vi "get Object By Name.vi"(10 "Name":string, 11 "Scene in":refnum<class "Scene.lvclass">) -> (2 "Index":i32, 3 "Object":T1 {"Triangles"."Vertex 3"."UV"."v" min=0 max=1 step=0.1; "Triangles"."Vertex 3"."UV"."u" min=0 max=1 step=0.1; "Triangles"."Vertex 2"."UV"."v" min=0 max=1 step=0.1; "Triangles"."Vertex 2"."UV"."u" min=0 max=1 step=0.1; "Triangles"."Vertex 1"."UV"."v" min=0 max=1 step=0.1; "Triangles"."Vertex 1"."UV"."u" min=0 max=1 step=0.1})   [LabVIEW 2020, in "Scene.lvclass"]
uses:
  Scene.lvclass
  Scene.lvclass/Scene.ctl
  Graphics/Libraries/3D/Vector 3D.ctl
  Graphics/Libraries/3D/3D.lvlib
  Graphics/Libraries/3D/Transform.ctl
  Graphics/Libraries/3D/Object.ctl
  Graphics/Libraries/Raster/UV.ctl
  Graphics/Libraries/Raster/Raster.lvlib
  Graphics/Libraries/3D/Vertex.ctl
  Graphics/Libraries/3D/Triangle.ctl
  Graphics/Libraries/Raster/Rectangle Dimensions.ctl
  Graphics/Libraries/Raster/Texture.ctl
  Graphics/Libraries/3D/Material.ctl
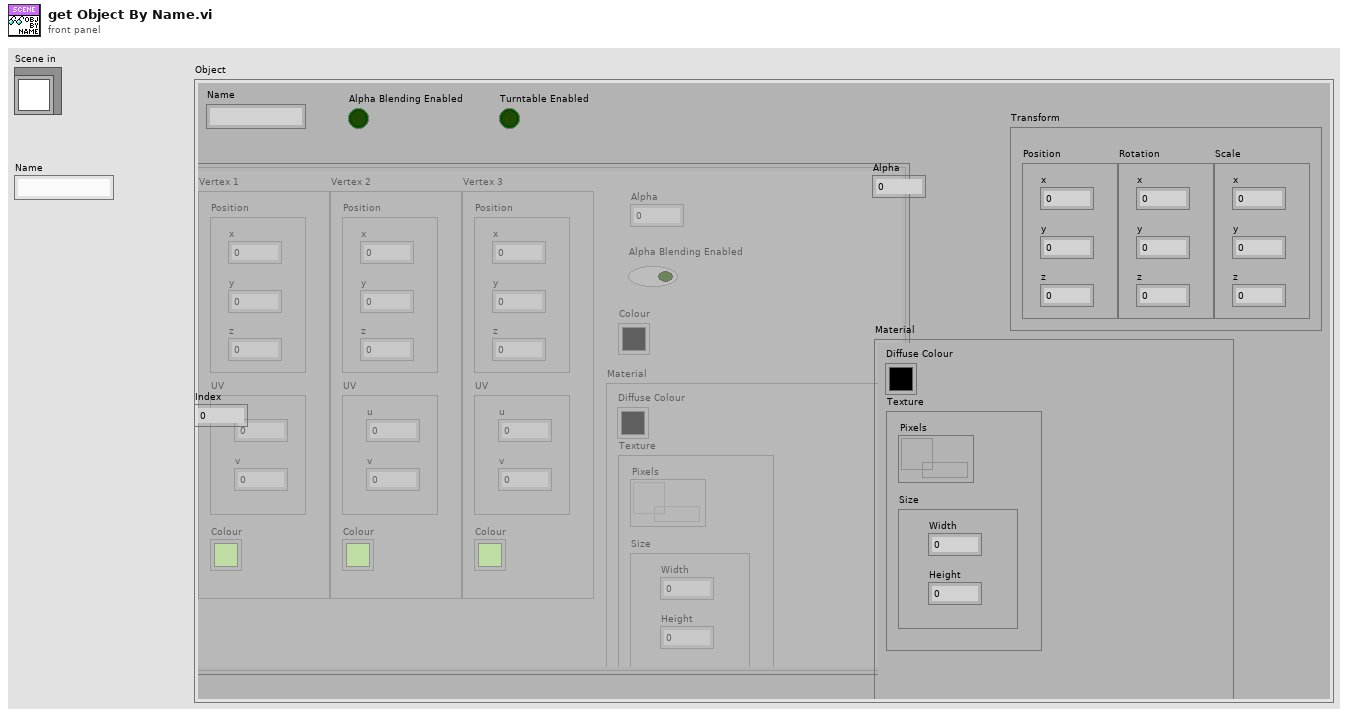
[diagram p1: front panel]
types:
  T1 = typedef "3D.lvlib/Object.ctl" = cluster{"Triangles":T2[], "Transform":T9, "Name":string, "Alpha Blending Enabled":bool, "Alpha":dbl, "Turntable Enabled":bool, "Material":T6}
  T2 = typedef "3D.lvlib/Triangle.ctl" = cluster{"Vertex 1":T3, "Vertex 2":T3, "Vertex 3":T3, "Alpha":dbl, "Alpha Blending Enabled":bool, "Colour":u32, "Material":T6}
  T3 = typedef "3D.lvlib/Vertex.ctl" = cluster{"Position":T4, "UV":T5, "Colour":u32}
  T4 = typedef "3D.lvlib/Vector 3D.ctl" = cluster{"x":sgl, "y":sgl, "z":sgl}
  T5 = typedef "Raster.lvlib/UV.ctl" = cluster{"u":sgl, "v":sgl}
  T6 = typedef "3D.lvlib/Material.ctl" = cluster{"Diffuse Colour":u32, "Texture":T7}
  T7 = typedef "Raster.lvlib/Texture.ctl" = cluster{"Pixels":refnum<data-value>, "Size":T8}
  T8 = typedef "Raster.lvlib/Rectangle Dimensions.ctl" = cluster{"Width":u32, "Height":u32}
  T9 = typedef "3D.lvlib/Transform.ctl" = cluster{"Position":T4, "Rotation":T4, "Scale":T4}
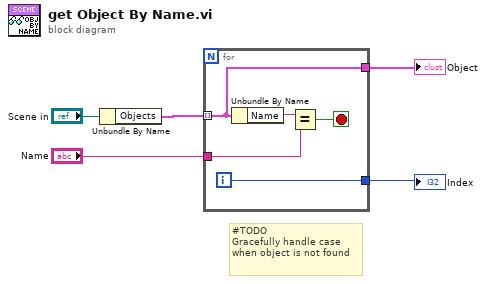
[diagram p0: block diagram]
diagram:
  # "#TODO\nGracefully handle case when object is not found"
  n1 = Unbundle By Name("Scene in") -> ("Objects"=w4:T1[])
  n2 = for {
    tunnel: w4 -> [w10] mode=indexing
    tunnel: [w10] -> w3
    tunnel: "Name" -> [w8]
    tunnel: [w6] -> w1
    i -> [w6]
    stop <- w7 stop-if-true
    n3 = Unbundle By Name(w10) -> ("Name"=w9:string)
    n4 = Equal?(x=w9, y=w8) -> (x = y?=w7:bool)
  }
  "Object" <- w3
  "Index" <- w1
